vi "IMAQdx Get Buffer Difference.vi"(10 "Previous Buffer Number":i32 format="%.0x", 11 "Current BufferNumber":i32) -> (3 "Buffer Difference":i32)   [LabVIEW 2020, in "NI_Vision_Acquisition_Software.lvlib"]
uses:
  NI_Vision_Acquisition_Software.lvlib
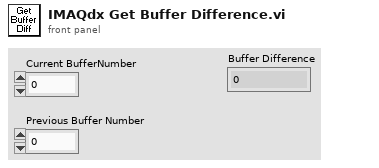
[diagram p1: front panel]
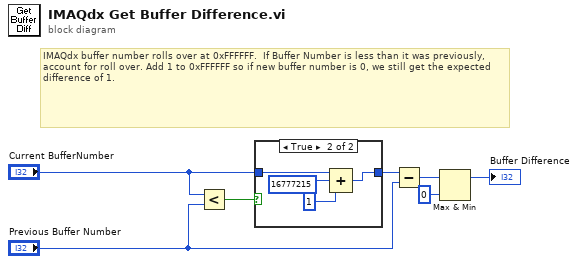
[diagram p0: block diagram]
diagram:
  # "IMAQdx buffer number rolls over at 0xFFFFFF.  If Buffer Number is less than it was previously, account for roll over. Add 1 to 0xFFFFFF so if new buffer number is 0, we still get the expected difference of 1."
  n1 = Less?(x="Current BufferNumber", y="Previous Buffer Number") -> (x < y?=w7:bool)
  n2 = case shown="True" w7 {
    tunnel: "Current BufferNumber" -> [w8 w12]
    tunnel: [w8 w9] -> w2
    frame False {
      # "No roll over"
    }
    frame True {
      n3 = Compound Arithmetic op=ADD(w12, 16777215 ("x"), 1 ("value")) -> (w9:i32)
    }
  }
  n4 = Subtract(x=w2, y="Previous Buffer Number") -> (x-y=w6:i32)
  n5 = Max & Min(x=w6, y=0) -> (max(x,y)=→"Buffer Difference":i32)  [unwired: 1 out]
